vi "Get Key Names.vi"(7 "section":string, 8 "error in (no error)":errorcluster, 11 "refnum":T1) -> (0 "error out":errorcluster, 1 "key names":string[](array[string]), 2 "section exists?":bool, 3 "refnum out":T1)   [LabVIEW 2017]
doc: "Gets the names of all keys in the specified section from the configuration data identified by <B>refnum</B>."
uses:
  DSFConfig.lvlib
  DSF Config Data RefNum.ctl
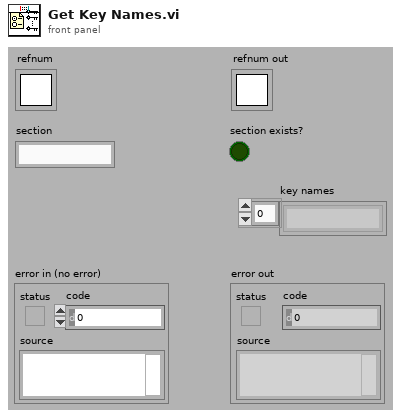
[diagram p1: front panel]
types:
  T1 = typedef "DSFConfig.lvlib/DSF Config Data RefNum.ctl" = refnum<k1>
  T2 = typedef "DSFConfig.lvlib/Config Queue.ctl" = refnum<queue>
  T3 = typedef "DSFConfig.lvlib/Config Data.ctl" = cluster{"dsf configuration":T4, "path":path, "dirty":bool}
  T4 = typedef "DSFConfig.lvlib/DSF Config.ctl" = cluster{"dsf":T5, "configuration":T5, "plugins":T6[], "groups":T9[], "transfers":T11[], "channels":T13[], "settings":T15[]}
  T5 = typedef "DSFConfig.lvlib/Version Info.ctl" = cluster{"major":u32, "minor":u32, "fix":u32, "build":string}
  T6 = typedef "DSFConfig.lvlib/DSF Plugin.ctl" = cluster{"id":string, "values":T7}
  T7 = typedef "DSFConfig.lvlib/DSF Plugin Info.ctl" = cluster{"type":string, "timing":T8, "group ids":string[], "settings id":string}
  T8 = typedef "DSFConfig.lvlib/DSF Timing Info.ctl" = cluster{"decimation":i32, "offset":i32}
  T9 = typedef "DSFConfig.lvlib/DSF Group.ctl" = cluster{"id":string, "values":T10}
  T10 = typedef "DSFConfig.lvlib/DSF Group Info.ctl" = cluster{"direction":i32, "timing":T8, "transfer ids":string[], "settings id":string}
  T11 = typedef "DSFConfig.lvlib/DSF Transfer.ctl" = cluster{"id":string, "values":T12}
  T12 = typedef "DSFConfig.lvlib/DSF Transfer Info.ctl" = cluster{"byte order":i32, "channel ids":string[], "settings id":string}
  T13 = typedef "DSFConfig.lvlib/DSF Channel.ctl" = cluster{"id":string, "values":T14}
  T14 = typedef "DSFConfig.lvlib/DSF Channel Info.ctl" = cluster{"count":i32, "offset":i32, "data type":i32, "resource path":string, "settings id":string}
  T15 = typedef "DSFConfig.lvlib/DSF Settings.ctl" = cluster{"id":string, "values":T16}
  T16 = typedef "DSFConfig.lvlib/DSF Settings Info.ctl" = cluster{"key":string, "value":string}[]
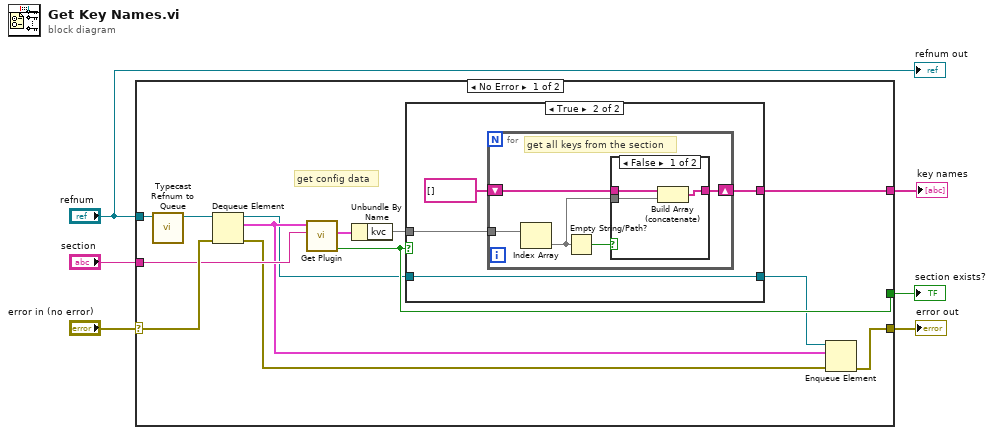
[diagram p0: block diagram]
diagram:
  n1 = case shown="No Error" "error in (no error)" {
    selector: "error in (no error)" -> [w16 w34]
    tunnel: [w13 _] -> w2
    tunnel: [w19 _] -> w1
    tunnel: [w10 w34] -> w4
    tunnel: "refnum" -> [w18 _]
    tunnel: "section" -> [w12 _]
    frame No Error {
      # "get config data"
      n2 = call "Typecast Refnum to Queue.vi"("refnum in"=w18) -> ("queue out"=w17:T2)  [unwired: 10 in]
      n3 = Dequeue Element(queue=w17, error in (no error)=w16) -> (queue out=w8:T2, element=w9:T3, error out=w11:errorcluster)  [unwired: 1 in, 1 out]
      n4 = call "Get Plugin.vi"("id"=w12, "element"=w9) -> ("exists?"=w13:bool, "info"=w15:T7)  [unwired: 6 in, 2 out]
      n5 = Unbundle By Name(w15) -> ("kvc"=w14)
      n6 = case shown="True" w13 {
        tunnel: [_ w23] -> w19
        tunnel: w14 -> [_ w24]
        tunnel: w8 -> [w20 w21]
        tunnel: [w20 w21] -> w7
        frame False {
        }
        frame True {
          n7 = for {
            tunnel: w24 -> [w29]
            shift-right: [w26] -> w23
            shift-left: string[] [] -> [w27]
            # "get all keys from the section"
            n8 = Index Array(array=w29) -> (element=w25)  [unwired: 1 in]
            n9 = Empty String/Path?(string/path=w25) -> (empty?=w28:bool)
            n10 = case shown="False" w28 {
              tunnel: w27 -> [w31 w33]
              tunnel: [w30 w33] -> w26
              tunnel: w25 -> [w32 _]
              frame False {
                n11 = Build Array (concatenate)(w31, w32) -> (w30:string[])
              }
              frame True {
              }
            }
          }
        }
      }
      n12 = Enqueue Element(queue=w7, element=w9, error in (no error)=w11) -> (error out=w10:errorcluster)  [unwired: 1 in, 2 out]
    }
    frame Error {
    }
  }
  "error out" <- w4
  "section exists?" <- w2
  "key names" <- w1
  "refnum out" <- "refnum"
